vi "test_TxUDP-RxUDP_Redundant.vi"(8 "error in":errorcluster, 11 "reference in":refnum<class "AIM ARINC 664 Loopback-MultiDevice.lvclass">) -> (0 "error out":errorcluster, 3 "reference out":refnum<class "AIM ARINC 664 Loopback-MultiDevice.lvclass">)   [LabVIEW 2020, in "AIM ARINC 664 Loopback-MultiDevice.lvclass"]
uses:
  AIM ARINC 664 Loopback-MultiDevice.lvclass
  C:/Program Files/National Instruments/LabVIEW 2024/vi.lib/NI/VeriStand Custom Device Testing Tools/VeriStandTestCase/VeriStandTestCase.lvclass
  AIM ARINC 664 Loopback-MultiDevice.lvclass/AIM ARINC 664 Loopback-MultiDevice.ctl
  b47c41b5-a02e-49d5-b852-4e28f097d7ad.vi
  6a3dd3ed-914d-4d14-bf18-724521aa5e28.vi
  8abe1e9f-12f7-4d29-bb0e-ea5e1950c3f4.vi
  NationalInstruments.VeriStand.SystemDefinitionAPI
  <vilib>/addons/_JKI Toolkits/VI Tester/TestCase.llb/TestCase.lvclass
  <vilib>/NI/VeriStand Custom Device Testing Tools/VeriStandTestCase/VeriStandTestCase.lvclass
  Scripting/AIM ARINC 664 Scripting.lvlib
  <vilib>/NI VeriStand/Custom Device API/Custom Device API.lvlib
  C:/Program Files/National Instruments/LabVIEW 2024/vi.lib/addons/_JKI Toolkits/VI Tester/TestCase.llb/TestCase.lvclass
panel:
  out "resulting string":string
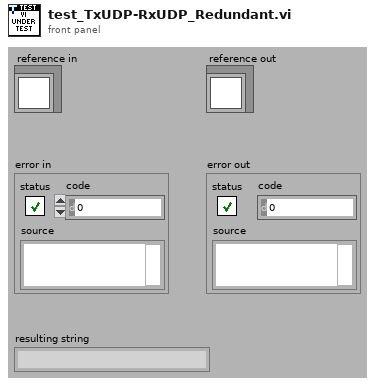
[diagram p1: front panel]
types:
  T1 = typedef "Custom Device API.lvlib/Custom Device Item Ref.ctl" = u64
  T2 = typedef "Custom Device API.lvlib/Custom Device Item Info.ctl" = cluster{"Name":string, "Is Channel":bool, "GUID":string, "Is Waveform":bool}
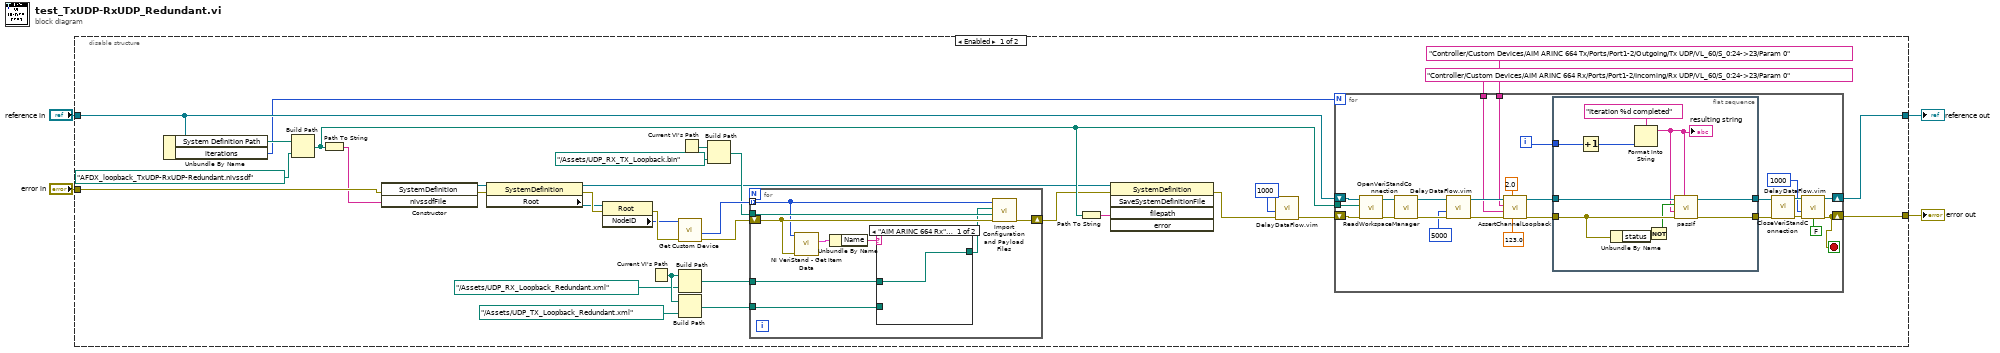
[diagram p0: block diagram]
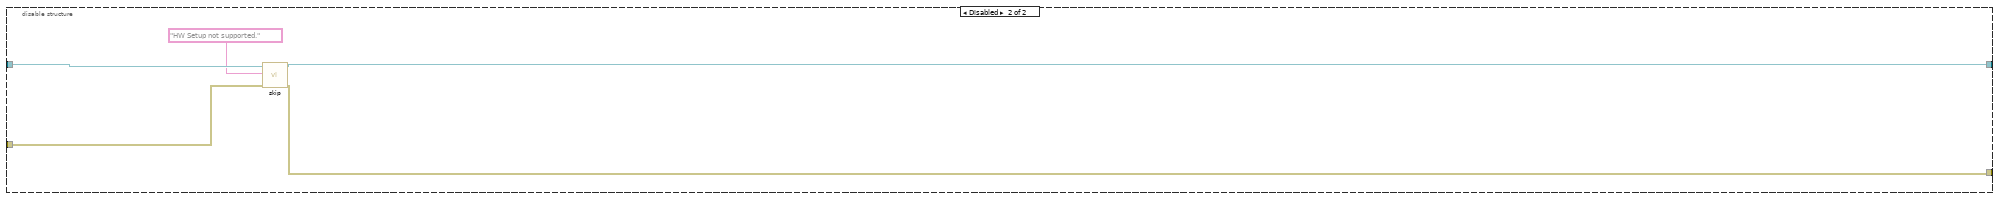
[diagram p3: hidden frame]
diagram:
  n1 = disable-structure shown="Enabled" {
    disable-tunnel: "reference in" -> [w37 w86]
    disable-tunnel: "error in" -> [w8 w85]
    disable-tunnel: [w34 w84] -> w2
    disable-tunnel: [w33 w83] -> w1
    frame Enabled {
      n2 = Unbundle By Name(w37) -> ("System Definition Path"=w36:path, "iterations"=w30:i32)
      n3 = Build Path(base path=w36, name or relative path=path "AFDX_loopback_TxUDP-RxUDP-Redundant.nivssdf") -> (appended path=w32:path)
      n4 = Path To String(path=w32) -> (string=w7:string)
      n5 = constructor class="SystemDefinition"(error in=w8, "nivssdfFile"=w7) -> (reference out=w12:refnum<k24>, error out=w14:errorcluster)  [unwired: 2 in, 2 out]
      n6 = property class="SystemDefinition"(reference=w12, error in=w14) -> (reference out=w5:refnum<k24>, error out=w15:errorcluster, "Root"=w13:refnum<k24>)
      n7 = property class="Root"(reference=w13, error in=w15) -> (error out=w19:errorcluster, "NodeID"=w18:u64)  [unwired: 1 out]
      n8 = Current VI's Path() -> (path=w22:path)
      n9 = call "Get Custom Device.vi"("error in"=w19, "custom device ref in"=w18) -> ("error out"=w20:errorcluster, "Item Refs"=w21:T1[])  [unwired: 5 in, 3 out]
      n10 = Build Path(base path=w22, name or relative path=path "../Assets/UDP_RX_Loopback_Redundant.xml") -> (appended path=w24:path)
      n11 = Build Path(base path=w22, name or relative path=path "../Assets/UDP_TX_Loopback_Redundant.xml") -> (appended path=w23:path)
      n12 = Current VI's Path() -> (path=w16:path)
      n13 = Build Path(base path=w16, name or relative path=path "../Assets/UDP_RX_TX_Loopback.bin") -> (appended path=w17:path)
      n14 = for {
        tunnel: w17 -> [w46]
        tunnel: w21 -> [w39] mode=indexing
        shift-right: [w45] -> w6
        shift-left: w20 -> [w44]
        tunnel: w23 -> [w40]
        tunnel: w24 -> [w38]
        n15 = call <vilib>:"NI VeriStand - Get Item Data.vi"("error in (no error)"=w44, "Item Ref in"=w39) -> ("Item Info"=w43:T2)  [unwired: 6 in, 3 out]
        n16 = Unbundle By Name(w43) -> ("Name"=w42:string)
        n17 = case shown="\"AIM ARINC 664 Rx\", Default" w42 {
          tunnel: [w47 w48] -> w41
          tunnel: w40 -> [_ w48]
          tunnel: w38 -> [w47 _]
          frame "AIM ARINC 664 Rx", Default {
          }
          frame "AIM ARINC 664 Tx" {
          }
        }
        n18 = call "Import Configuration and Payload Files.vi"("error in"=w44, "payload file path"=w46, "parameters configuration file path"=w41, "custom device ref"=w39) -> ("error out"=w45:errorcluster)  [unwired: 6 in, 1 out]
      }
      n19 = Path To String(path=w32) -> (string=w31:string)
      n20 = invoke class="SystemDefinition" method="SaveSystemDefinitionFile"(reference=w5, error in=w6, "filepath"=w31) -> (error out=w29:errorcluster)  [unwired: 2 in, 4 out]
      n21 = call "DelayDataFlow.vim"("value in"=w29, "milliseconds to wait"=u32 1000) -> ("value out"=w28:errorcluster)  [unwired: 2 in, 1 out]
      n22 = for {
        N: w30 -> [_]
        tunnel: w32 -> [w64]
        shift-right: [w69] -> w33
        shift-left: w37 -> [w71]
        shift-right: [w49] -> w34
        shift-left: w28 -> [w65]
        tunnel: "Controller/Custom Devices/AIM ARINC 664 Rx/Ports/Port1-2/Incoming/Rx UDP/VL_60/S_0:24->23/Param 0" -> [w51]
        tunnel: "Controller/Custom Devices/AIM ARINC 664 Tx/Ports/Port1-2/Outgoing/Tx UDP/VL_60/S_0:24->23/Param 0" -> [w50]
        i -> [w53]
        stop <- w49 stop-if-true
        n23 = call-dynamic "OpenVeriStandConnection.vi"("error in (no error)"=w65, "System Definition File"=w64, "VeriStand Test Case in"=w71) -> ("error out"=w70:errorcluster, "VeriStand Test Case out"=w68:refnum<class "AIM ARINC 664 Loopback-MultiDevice.lvclass">)  [unwired: 6 in, 1 out]
        n24 = call-dynamic "ReadWorkspaceManager.vi"("error in (no error)"=w70, "VeriStand Test Case in"=w68) -> ("error out"=w67:errorcluster, "VeriStand Test Case out"=w62:refnum<class "AIM ARINC 664 Loopback-MultiDevice.lvclass">)  [unwired: 7 in, 1 out]
        n25 = call "DelayDataFlow.vim"("value in"=w67, "milliseconds to wait"=u32 5000) -> ("value out"=w63:errorcluster)  [unwired: 2 in, 1 out]
        n26 = call <vilib>:"AssertChannelLoopback.vi"("Value"=123.0, "Timeout (1 second)"=2.0, "error in (no error)"=w63, "Read Channel"=w51, "Write Channel"=w50, "VeriStand Test Case in"=w62) -> ("error out"=w54:errorcluster, "VeriStand Test Case out"=w52:refnum<class "AIM ARINC 664 Loopback-MultiDevice.lvclass">)  [unwired: 4 in]
        n27 = flat-sequence {
          tunnel: [w81] -> w56
          tunnel: [w80] -> w55
          tunnel: w54 -> [w79]
          tunnel: w53 -> [w75]
          tunnel: w52 -> [w73]
          frame #0 {
            n28 = Increment(x=w75) -> (x+1=w74:i32)
            n29 = Unbundle By Name(w79) -> ("status"=w78:bool)
            n30 = Format Into String(format string="Iteration %d completed", w74) -> (resulting string=w72:string)  [unwired: 2 in, 1 out]
            "resulting string" <- w72
            n31 = Not(x=w78) -> (.not. x?=w77:bool)
            n32 = call-dynamic "passIf.vi"("custom report message (\"\")"=w72, "error in (no error)"=w79, "message (\"\")"=w72, "pass"=w77, "TestCase in"=w73) -> ("error out"=w80:errorcluster, "TestCase out"=w81:refnum<class "AIM ARINC 664 Loopback-MultiDevice.lvclass">)  [unwired: 5 in]
          }
        }
        n33 = call-dynamic "CloseVeriStandConnection.vi"("error in (no error)"=w55, "VeriStand Test Case in"=w56) -> ("error out"=w59:errorcluster, "VeriStand Test Case out"=w69:refnum<class "AIM ARINC 664 Loopback-MultiDevice.lvclass">)  [unwired: 8 in]
        n34 = call "DelayDataFlow.vim"("value in"=w59, "milliseconds to wait"=u32 1000, "no delay on error (T)"=FALSE) -> ("value out"=w49:errorcluster)  [unwired: 1 in, 1 out]
      }
    }
    frame Disabled {
      n35 = call <vilib>:"skip.vi"("error in (no error)"=w85, "skipMessage"="HW Setup not supported.", "TestCase in"=w86) -> ("error out"=w84:errorcluster, "TestCase out"=w83:refnum<class "AIM ARINC 664 Loopback-MultiDevice.lvclass">)  [unwired: 7 in]
    }
  }
  "error out" <- w2
  "reference out" <- w1
